vi "Set Slit Speed.vi"(7 "Mono System # (0)":T2, 8 "error in (no error)":errorcluster, 9 "Frequency":dbl[unit], 10 "Slit (Front/Axial Entrance)":T1, 11 "VISA resource name":refnum<visa-resource-name>) -> (0 "error out":errorcluster, 3 "VISA resource name out":refnum<visa-resource-name>)   [LabVIEW 2009, in "JY-SPEX-TRIAX.lvlib"]
doc: "Sets the rate at which the slits will move."
uses:
  JY-SPEX-TRIAX.lvlib
  controls.llb/Monochromator System Number.ctl
  controls.llb/Slits.ctl
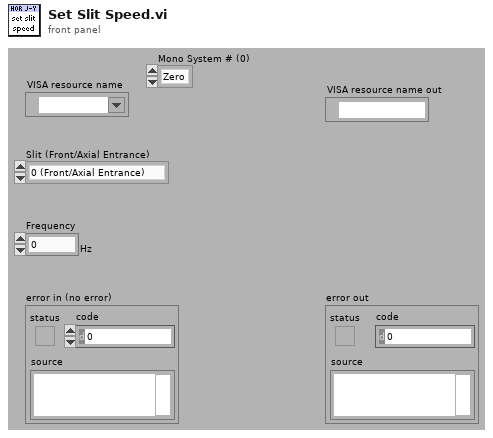
[diagram p1: front panel]
types:
  T1 = typedef "JY-SPEX-TRIAX.lvlib/Slits.ctl" = enum16{"0 (Front/Axial Entrance)", "1 (Side/Lateral Entrance)", "2 (Front/Axial Exit)", "3 (Side/Lateral Exit)"}
  T2 = typedef "JY-SPEX-TRIAX.lvlib/Monochromator System Number.ctl" = enum16{"Zero", "One"}
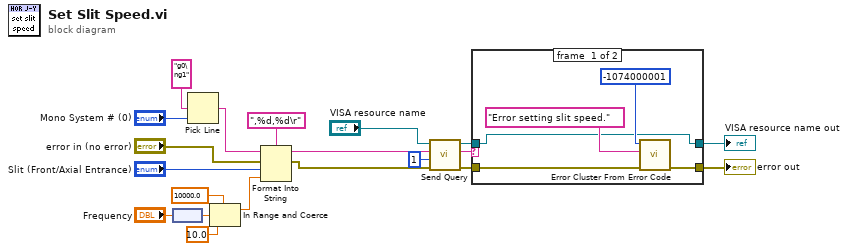
[diagram p0: block diagram]
diagram:
  n1 = node("Frequency") -> (w19:dbl)
  n2 = Pick Line(multi-line string="g0\ng1", line index="Mono System # (0)") -> (output string=w14:string)  [unwired: 1 out]
  n3 = In Range and Coerce(upper limit=10000.0, x=w19, lower limit=10.0) -> (coerced(x)=w12:dbl)  [unwired: 1 out]
  n4 = Format Into String(format string=",%d,%d\r", initial string=w14, error in="error in (no error)", "Slit (Front/Axial Entrance)", w12) -> (resulting string=w11:string, error out=w8:errorcluster)
  n5 = call "Send Query.vi"("error in (no error)"=w8, "byte count"=u32 1, "write buffer"=w11, "VISA resource name"="VISA resource name") -> ("error out"=w3:errorcluster, "read buffer"=w6:string, "VISA resource name out"=w5:refnum<visa-resource-name>)  [unwired: 5 out]
  n6 = case shown="Default" w6 {
    tunnel: w5 -> [w21 w27]
    tunnel: [w21 w27] -> w4
    tunnel: w3 -> [w23 w26]
    tunnel: [w22 w26] -> w2
    frame #0 {
      n7 = call <vilib>:"Error Cluster From Error Code.vi"("error in (no error)"=w23, "error message (\"\")"="Error setting slit speed." ("error message (\"\")"), "error code (0)"=-1074000001) -> ("error out"=w22:errorcluster)  [unwired: 1 in, 5 out]
    }
    frame #1 {
    }
  }
  "VISA resource name out" <- w4
  "error out" <- w2
